vi "Peaks Scatter Plot v2.vi"(0 "Host Plot Controls":T1={"refresh"=FALSE, "PMTs for Host"={"Sa"=0, "Sb"=1, "g-factor"=1}, "Peaks"={"# bins"=1000, "min"=0.020751953125, "max"=0.00103759765625}, "Averages"={"# bins"=1000, "max"=0.020751953125, "min"=0.00103759765625}, "Durations"={"# bins"=1000, "max"=20.0, "min"=8.0}, "FP-FPGA"={"# bins"=1000, "max"=20.0, "min"=8.0}, "FP-Host"={"# bins"=1000, "max"=20.0, "min"=8.0}, "Sort Mode"=0} {"Sort Mode" items=["Peak Max", "Peak Average"]}, 1 "number to display":i32=10000, 7 "peaks data":T2, 12 "?":cluster{dbl[], dbl[], dbl[], dbl[]}={array[1000 elements], array[1000 elements], array[1000 elements], array[1000 elements]}) -> (4 "scatter":cluster{"Max1":dbl[], "Max1":dbl[]}[](graph), 14 "?":cluster{dbl[], dbl[], dbl[], dbl[]})   [LabVIEW 2009]
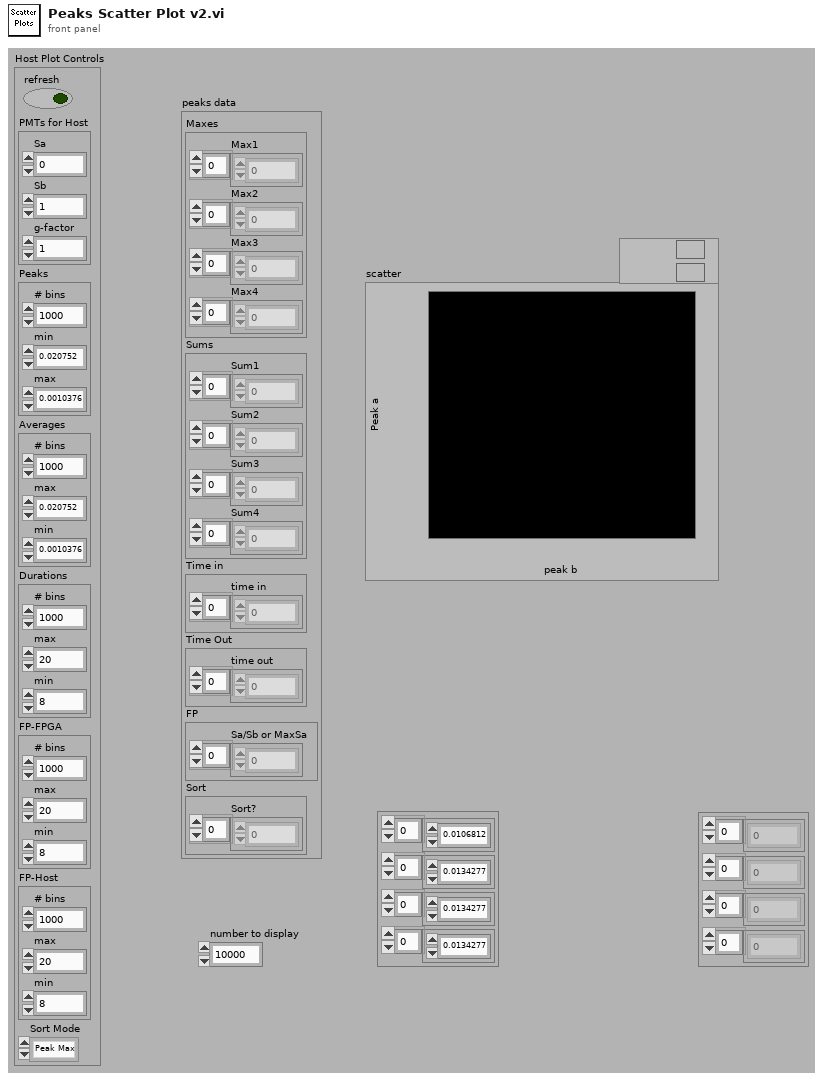
[diagram p1: front panel]
types:
  T1 = cluster{"refresh":bool, "PMTs for Host":cluster{"Sa":i8, "Sb":i8, "g-factor":i32}, "Peaks":cluster{"# bins":i32, "min":dbl, "max":dbl}, "Averages":cluster{"# bins":i32, "max":dbl, "min":dbl}, "Durations":cluster{"# bins":i32, "max":dbl, "min":dbl}, "FP-FPGA":cluster{"# bins":i32, "max":dbl, "min":dbl}, "FP-Host":cluster{"# bins":i32, "max":dbl, "min":dbl}, "Sort Mode":i8}
  T2 = cluster{"Maxes":cluster{"Max1":dbl[], "Max2":dbl[], "Max3":dbl[], "Max4":dbl[]}, "Sums":cluster{"Sum1":dbl[], "Sum2":dbl[], "Sum3":dbl[], "Sum4":dbl[]}, "Time in":cluster{"time in":dbl[]}, "Time Out":cluster{"time out":dbl[]}, "FP":cluster{"Sa/Sb or MaxSa":dbl[]}, "Sort":cluster{"Sort?":dbl[]}}
  T3 = cluster{"Sum1":dbl[], "Sum2":dbl[], "Sum3":dbl[], "Sum4":dbl[]}
  T4 = cluster{"Max1":dbl[], "Max2":dbl[], "Max3":dbl[], "Max4":dbl[]}
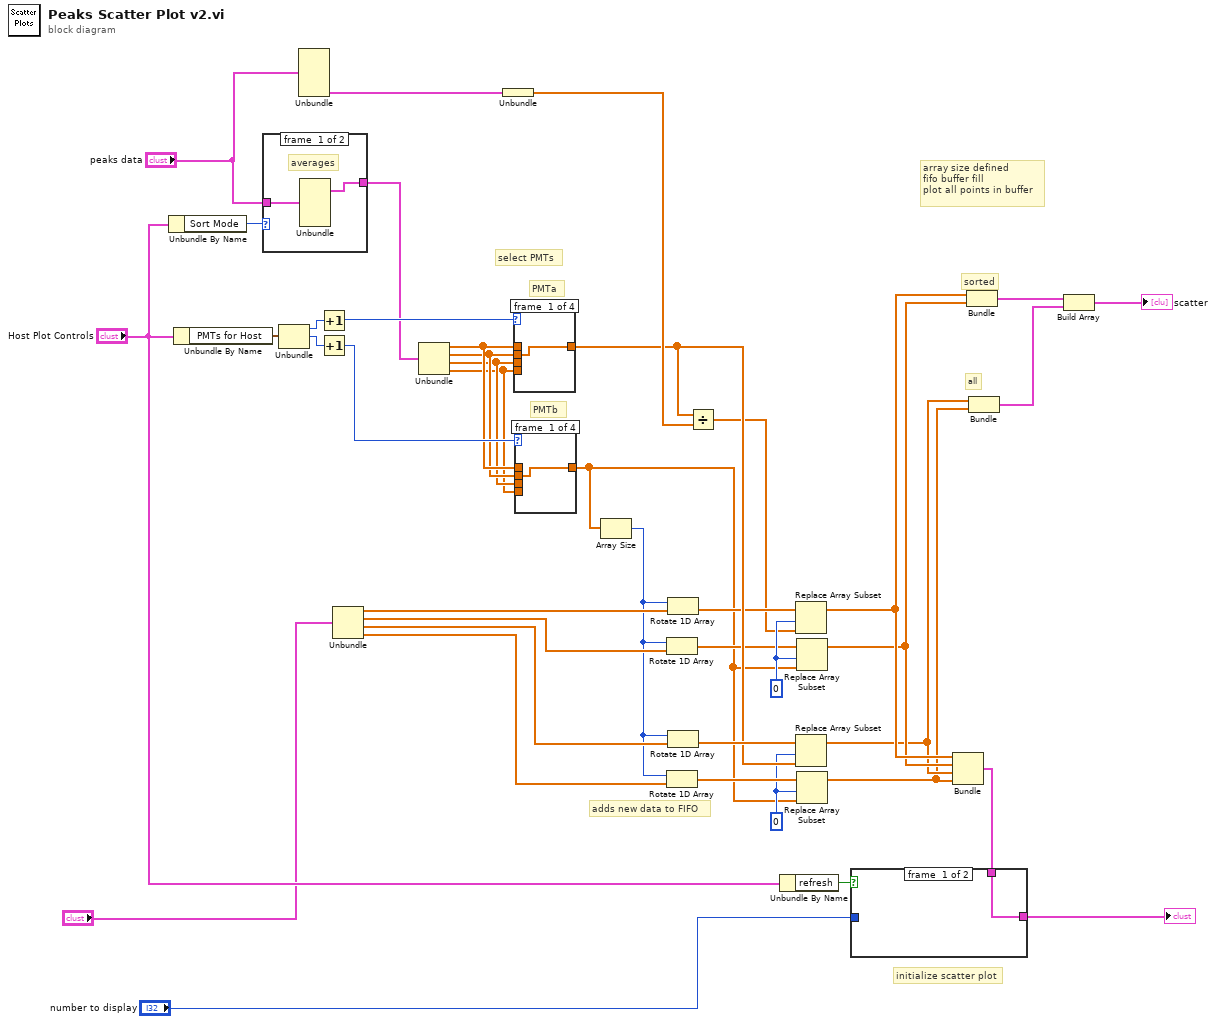
[diagram p0: block diagram]
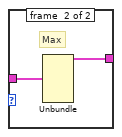
[diagram p2: hidden frame]
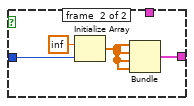
[diagram p3: hidden frame]
diagram:
  w16 = 0 ("index")
  w18 = 0 ("index")
  # "select PMTs"
  # "initialize scatter plot"
  # "adds new data to FIFO"
  # "array size defined\nfifo buffer fill\nplot all points in buffer"
  # "sorted"
  # "all"
  # "PMTb"
  # "PMTa"
  n1 = Unbundle By Name("Host Plot Controls") -> ("Sort Mode"=w25:i8)
  n2 = Unbundle By Name("Host Plot Controls") -> ("PMTs for Host"=w33:cluster{"Sa":i8, "Sb":i8, "g-factor":i32})
  n3 = case shown="0, Default" w25 {
    tunnel: "peaks data" -> [w43 w45]
    tunnel: [w42 w44] -> w27
    frame #0 {
      # "averages"
      n4 = Unbundle(w43) -> ("Sums"=w42:T3)  [unwired: 5 out]
    }
    frame #1 {
      # "Max"
      n5 = Unbundle(w45) -> ("Maxes"=w44:T4)  [unwired: 5 out]
    }
  }
  n6 = Unbundle(w33) -> ("Sa"=w39:i8, "Sb"=w38:i8)  [unwired: 1 out]
  n7 = Unbundle("peaks data") -> ("Sort"=w32:cluster{"Sort?":dbl[]})  [unwired: 5 out]
  n8 = Increment(x=w39) -> (x+1=w40:i8)
  n9 = Increment(x=w38) -> (x+1=w41:i8)
  n10 = Unbundle("?") -> (w12:dbl[], w11:dbl[], w10:dbl[], w9:dbl[])
  n11 = Unbundle(w27) -> ("Max1"=w37:dbl[], "Max2"=w36:dbl[], "Max3"=w35:dbl[], "Max4"=w34:dbl[])
  n12 = Unbundle(w32) -> ("Sort?"=w30:dbl[])
  n13 = case shown="1, Default" w40 {
    tunnel: w37 -> [_ _ _ w49]
    tunnel: w36 -> [w46 _ _ _]
    tunnel: w35 -> [_ w47 _ _]
    tunnel: w34 -> [_ _ w48 _]
    tunnel: [w46 w47 w48 w49] -> w19
    frame #0 {
    }
    frame #1 {
    }
    frame #2 {
    }
    frame #3 {
    }
  }
  n14 = case shown="1, Default" w41 {
    tunnel: w37 -> [_ _ _ w53]
    tunnel: w36 -> [w50 _ _ _]
    tunnel: w35 -> [_ w51 _ _]
    tunnel: w34 -> [_ _ w52 _]
    tunnel: [w50 w51 w52 w53] -> w7
    frame #0 {
    }
    frame #1 {
    }
    frame #2 {
    }
    frame #3 {
    }
  }
  n15 = Array Size(array=w7) -> (size(s)=w6:i32)
  n16 = Rotate 1D Array(1:w11, 2:w6) -> (0:w15:dbl[])
  n17 = Rotate 1D Array(1:w9, 2:w6) -> (0:w20:dbl[])
  n18 = Rotate 1D Array(1:w12, 2:w6) -> (0:w14:dbl[])
  n19 = Rotate 1D Array(1:w10, 2:w6) -> (0:w21:dbl[])
  n20 = Divide(x=w19, y=w30) -> (x/y=w8:dbl[])
  n21 = Unbundle By Name("Host Plot Controls") -> ("refresh"=w29:bool)
  n22 = Replace Array Subset(array=w14, new element=w8, index=w16) -> (w5:dbl[])
  n23 = Replace Array Subset(array=w21, new element=w19, index=w18) -> (w3:dbl[])
  n24 = Replace Array Subset(array=w15, new element=w7, index=w16) -> (w4:dbl[])
  n25 = Replace Array Subset(array=w20, new element=w7, index=w18) -> (w2:dbl[])
  n26 = Bundle(w5, w4, w3, w2) -> (w17:cluster{dbl[], dbl[], dbl[], dbl[]})  [unwired: 1 in]
  n27 = case shown="True" w29 {
    tunnel: w17 -> [w54 _]
    tunnel: [w54 w56] -> w13
    tunnel: "number to display" -> [_ w55]
    frame #0 {
    }
    frame #1 {
      n28 = Initialize Array(inf ("element"), w55) -> (w57:dbl[])
      n29 = Bundle(w57, w57, w57, w57) -> (w56:cluster{dbl[], dbl[], dbl[], dbl[]})  [unwired: 1 in]
    }
  }
  "?" <- w13
  n30 = Bundle(w5, w4) -> (w23:cluster{dbl[], dbl[]})  [unwired: 1 in]
  n31 = Bundle(w3, w2) -> (w22:cluster{dbl[], dbl[]})  [unwired: 1 in]
  n32 = Build Array(w23, w22) -> (→"scatter":cluster{dbl[], dbl[]}[])
